vi "Generate report graphs.vi"(8 "error in (no error)":errorcluster, 9 "Test Energies":dbl[](array[numeric]), 10 "report file path":path, 11 "file path":path) -> (0 "error out":errorcluster)   [LabVIEW 2015]
uses:
  <vilib>/addons/_office/word.llb/Word Easy Table (num).vi
  <vilib>/Utility/NIReport.llb/NI_report.lvclass
  <vilib>/Utility/NIReport.llb/Word/NI_Word.lvclass
  <vilib>/addons/_office/NI_ReportGenerationToolkit.lvlib
panel:
  out "Min and Max Temperatures":dbl[][](array[numeric])
  out "Full Shot - Discharge Voltage (V) and Current (A) against Time (s)":waveform(dbl)[](graph)
  out "Single Pulse - Discharge Voltage (V) and Current (A) against Time (ms)":waveform(dbl)[](graph)
  out "Temperature (Degrees C) against Time (s)":waveform(dbl)(graph)
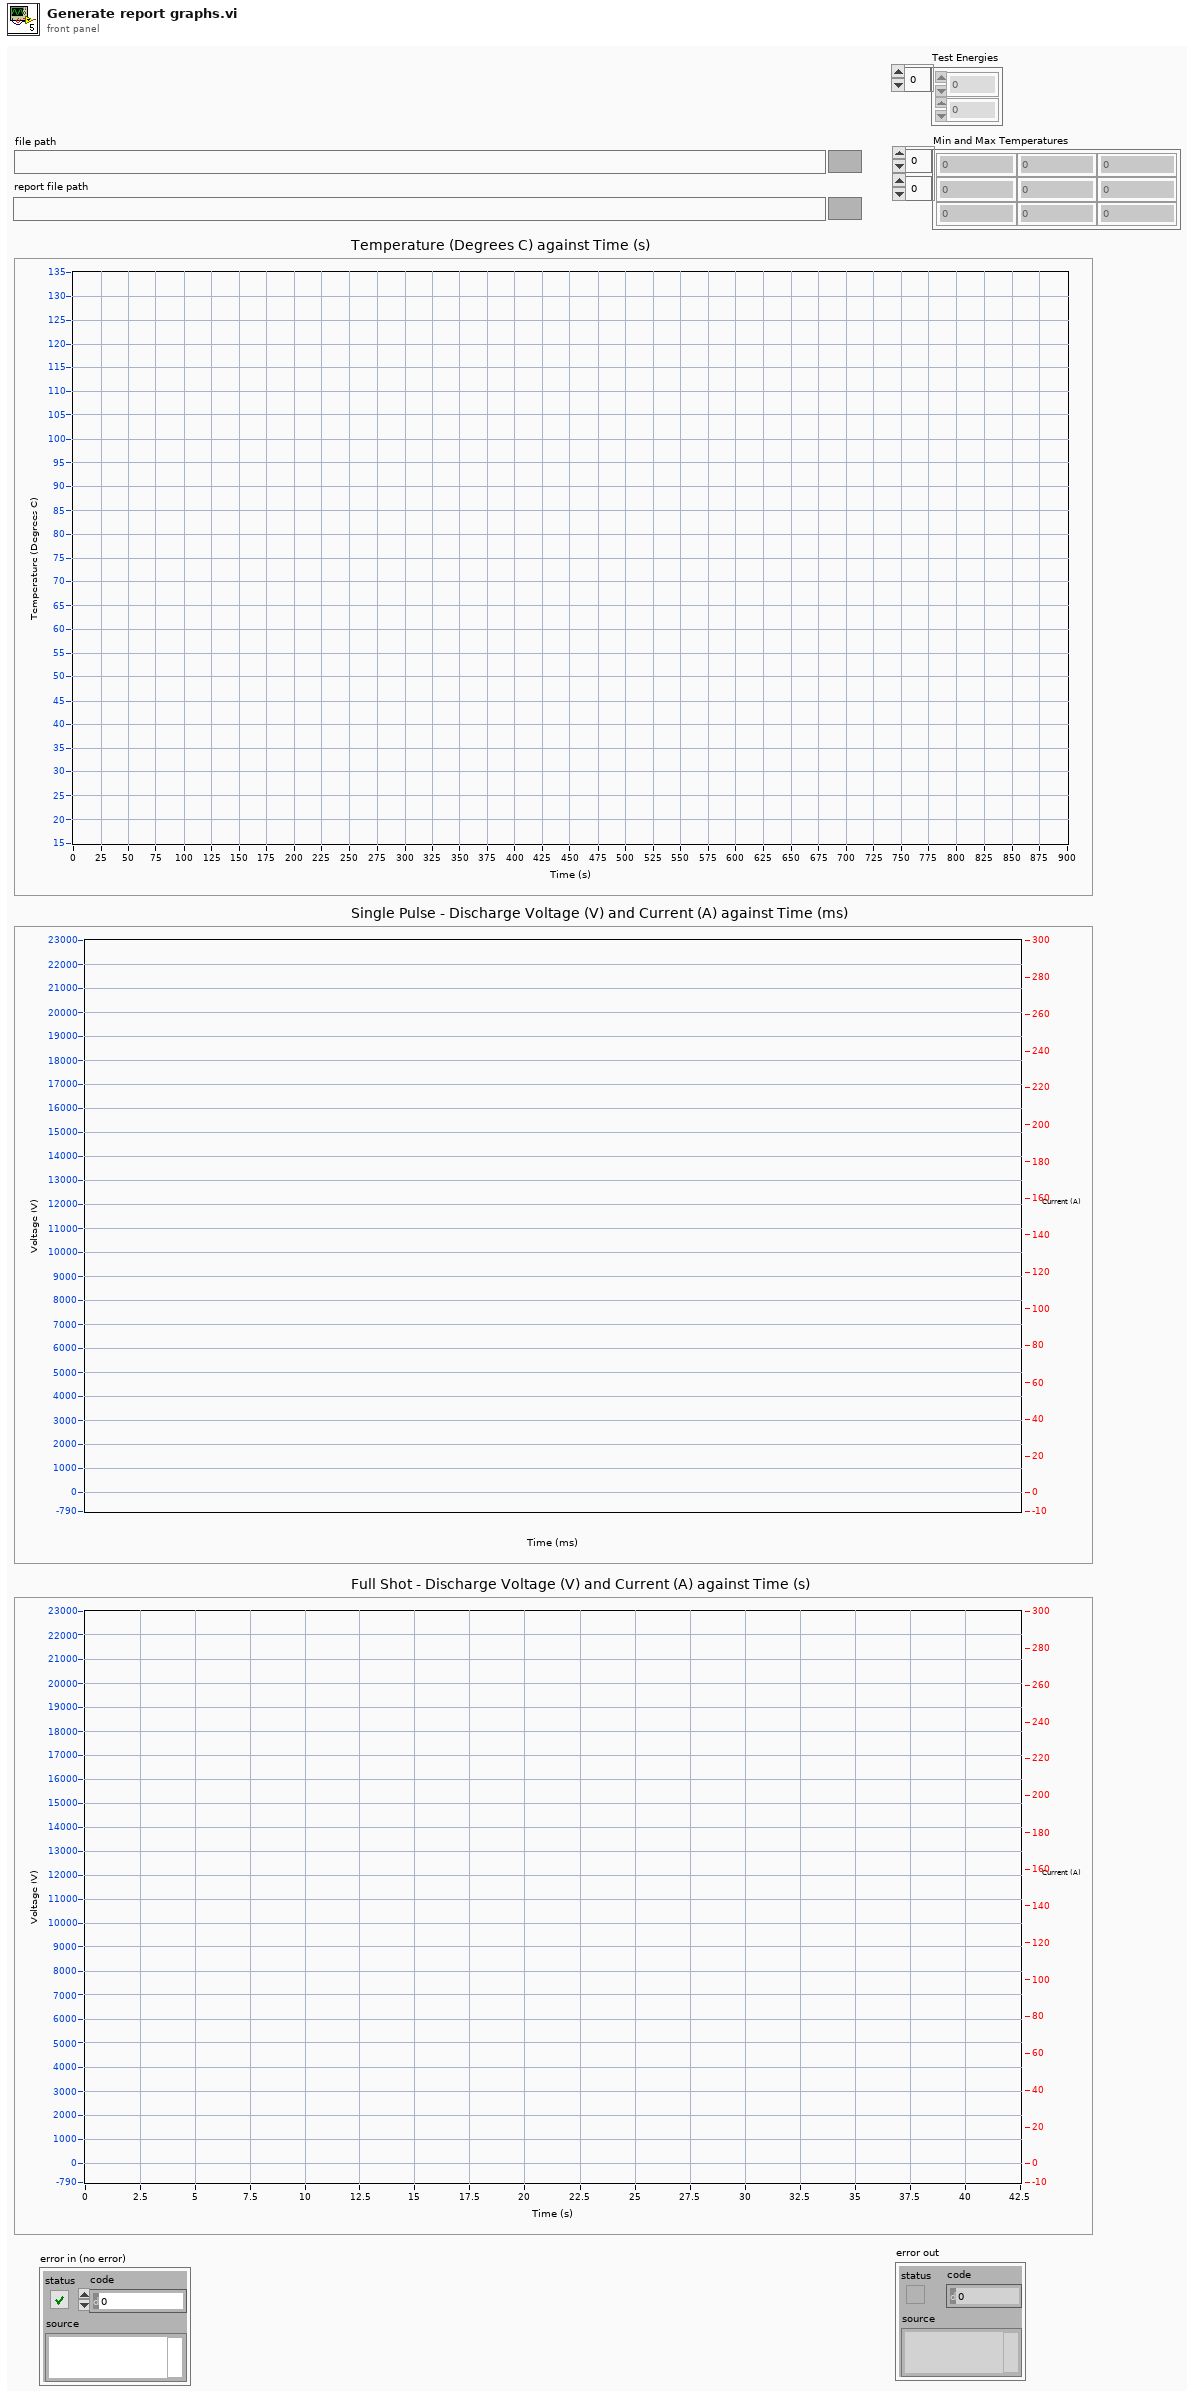
[diagram p1: front panel]
types:
  T1 = enum16{"Standard Report", "HTML", "Word", "Excel"}
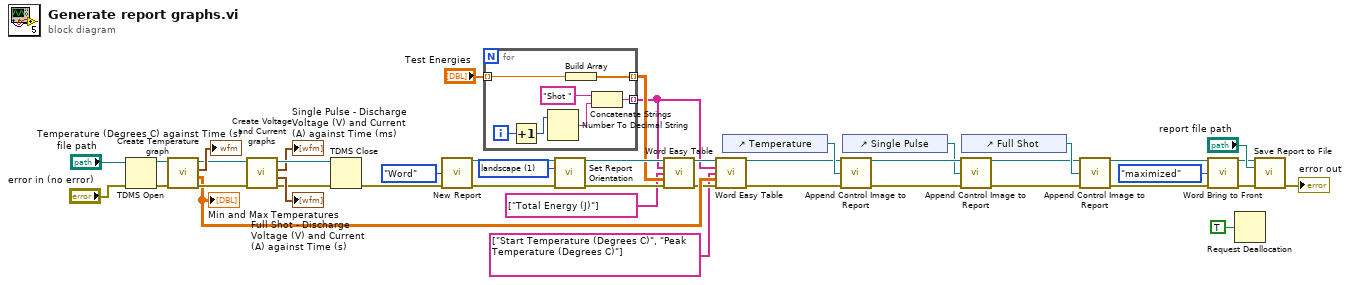
[diagram p0: block diagram]
diagram:
  w39 = 1 items=["portrait", "landscape"] ("orientation (portrait)")
  n1 = TDMS Open(8:"error in (no error)", 11:"file path") -> (0:w37:errorcluster, 3:w36:refnum<k34>)  [unwired: 5 in]
  n2 = call "Create Temperature graph.vi"("error in (no error)"=w37, "Refnum in"=w36) -> ("error out"=w30:errorcluster, "Min and Max Temperatures"=w6:dbl[][], "Waveform"=→"Temperature (Degrees C) against Time (s)":waveform(dbl), "Refnum out"=w34:refnum<k34>)  [unwired: 6 in]
  "Min and Max Temperatures" <- w6
  n3 = call "Create Voltage and Current graphs.vi"("error in (no error)"=w30, "Refnum in"=w34) -> ("error out"=w29:errorcluster, "Full Shot"=→"Full Shot - Discharge Voltage (V) and Current (A) against Time (s)":waveform(dbl)[], "Single Pulse"=→"Single Pulse - Discharge Voltage (V) and Current (A) against Time (ms)":waveform(dbl)[], "Refnum out"=w33:refnum<k34>)  [unwired: 6 in]
  n4 = TDMS Close(8:w29, 11:w33) -> (0:w28:errorcluster)  [unwired: 1 out]
  n5 = call <vilib>:"New Report.vi"("report type"=T1."Word", "error in (no error)"=w28) -> ("report out"=w41:refnum<class "NI_report.lvclass">, "error out"=w40:errorcluster)  [unwired: 12 in]
  n6 = for {
    tunnel: "Test Energies" -> [w47] mode=indexing
    tunnel: [w48] -> w3 mode=indexing
    tunnel: [w46] -> w10 mode=indexing
    i -> [w45]
    n7 = Increment(x=w45) -> (x+1=w44:i32)
    n8 = Number To Decimal String(number=w44) -> (decimal integer string=w49:string)  [unwired: 1 in]
    n9 = Build Array(w47) -> (w46:dbl[])
    n10 = Concatenate Strings("Shot ", w49) -> (w48:string)
  }
  n11 = call-dynamic "Set Report Orientation.vi"("report in"=w41, "orientation (portrait)"=w39, "error in (no error)"=w40) -> ("report out"=w12:refnum<class "NI_report.lvclass">, "error out"=w13:errorcluster)  [unwired: 11 in]
  n12 = call-poly <vilib>:"Word Easy Table.vi"("report in"=w12, "row headers"=w3, "column headers"=string[] ["Total Energy (J)"], "text data"=w10, "error in (no error)"=w13) -> ("report out"=w4:refnum<class "NI_report.lvclass">, "error out"=w5:errorcluster)  [unwired: 8 in, 1 out]
  n13 = call-poly <vilib>:"Word Easy Table.vi"("report in"=w4, "row headers"=w3, "column headers"=string[] ["Start Temperature (Degrees C)", "Peak Temperature (Degrees C)"], "text data"=w6, "error in (no error)"=w5) -> ("report out"=w8:refnum<class "NI_report.lvclass">, "error out"=w7:errorcluster)  [unwired: 8 in, 1 out]
  n14 = control-ref of="Temperature"() -> (w27:refnum<vi>)
  n15 = call-dynamic "Append Control Image to Report.vi"("report in"=w8, "ctrl reference"=w27, "error in (no error)"=w7) -> ("report out"=w26:refnum<class "NI_report.lvclass">, "error out"=w25:errorcluster)  [unwired: 9 in, 2 out]
  n16 = control-ref of="Single Pulse"() -> (w24:refnum<vi>)
  n17 = call-dynamic "Append Control Image to Report.vi"("report in"=w26, "ctrl reference"=w24, "error in (no error)"=w25) -> ("report out"=w22:refnum<class "NI_report.lvclass">, "error out"=w21:errorcluster)  [unwired: 9 in, 2 out]
  n18 = control-ref of="Full Shot"() -> (w23:refnum<vi>)
  n19 = call-dynamic "Append Control Image to Report.vi"("report in"=w22, "ctrl reference"=w23, "error in (no error)"=w21) -> ("report out"=w18:refnum<class "NI_report.lvclass">, "error out"=w17:errorcluster)  [unwired: 9 in, 2 out]
  n20 = call <vilib>:"Word Bring to Front.vi"("report in"=w18, "window state (maximized)"=enum16{"maximized", "minimized", "normal"}."maximized", "error in (no error)"=w17) -> ("report out"=w20:refnum<class "NI_report.lvclass">, "error out"=w19:errorcluster)  [unwired: 11 in]
  n21 = Request Deallocation(TRUE ("flag")) -> ()
  n22 = call-dynamic "Save Report to File.vi"("report in"=w20, "report file path"="report file path", "error in (no error)"=w19) -> ("error out"=→"error out":errorcluster)  [unwired: 11 in, 1 out]
